vi "JitterVCOLO.vi"() -> ()   [LabVIEW 2009]
uses:
  <vilib>/Analysis/4window.llb/windowTd.ctl
  <vilib>/measure/maspectr.llb/FFT Spectrum (Mag-Phase) for 1 Chan.vi
  <vilib>/measure/maspectr.llb/FFT Power Spectrum for 1 Chan.vi
  <vilib>/measure/macond.llb/FIR Filter for 1 Chan.vi
  <vilib>/ptbypt/NI_PtbyPt.lvlib
  <vilib>/measure/NI_MAPro.lvlib
  <vilib>/Analysis/NI_AALPro.lvlib
  <vilib>/measure/NI_MABase.lvlib
panel:
  in  "FFT View":T1={"dB On (F)"=TRUE, "unwrap phase (F)"=FALSE, "convert to degree (F)"=FALSE}
  out "VCO Period":ext=1.25000000000000000005e-7 format="%#_6p"
  out "LO Period":ext=1.6666666666666666666e-7 format="%#_6p"
  out "Equivalent LO RMS time jitter":ext format="%#_6p"
  out "Equivalent VCO RMS time jitter":ext=1.9894367886486917747e-10 format="%#_6p"
  in  "Sampling rate and number of samples to generate":cluster{"Fs":dbl, "#s":dbl}={"Fs"=40000000.0, "#s"=400000.0} {"Fs" format="%.2p"}
  out "df (Hz)":dbl=100.0
  out "averages completed":dbl=1.0
  in  "averaging parameters":T2={"averaging mode"=enum."RMS averaging", "weighting mode"=enum."Exponential", "number of averages"=20} {"number of averages" min=1}
  in  "optional FIR filter specifications":T3={"PB Gain"=0.0, "SB Gain"=-300.0, "Scale"=TRUE, "Window"=enum."Flat Top"} {"SB Gain" format="%.2p"; "PB Gain" format="%.2p"}
  out "Computed Cycles":i32=400000
  in  "Low Side / High Side":bool
  out "Phase Noise":cluster{"f0":dbl, "df":dbl, "magnitude":dbl[]}(graph)={"f0"=0.0, "df"=100.0, "magnitude"=[]}
  out "RF input":cluster{"f0":dbl, "df":dbl, "magnitude":dbl[]}(graph)={"f0"=0.0, "df"=99.74415623924635, "magnitude"=[]}
  in  "VCO power (dBm)":dbl
  in  "LO power (dBm)":dbl
  in  "RMS Phase Jitter VCO (Radians)":ext=0.01
  in  "RMS Phase Jitter LO (Radians)":ext
  in  "VCO  Frequency":ext=8000000.0 format="%#.6p"
  in  "IF Frequency":ext=2000000.0 format="%#.6p"
  # "Phase noise power spectum (dBc), only good out to the lower PB of the FIR filter used after the\nI/Q downconversion from the intermediate frequency step"
  # "Nyquist demands that Fs > 2 * (2 * VCO - IF) for Low Side,\nand Fs > 2 * (2 * VCO + IF) for High Side"
  # "Enter the number of samples to generate here. This will affect your\nfrequency granularity. More samples, more granularity. df = Fs / (#s)"
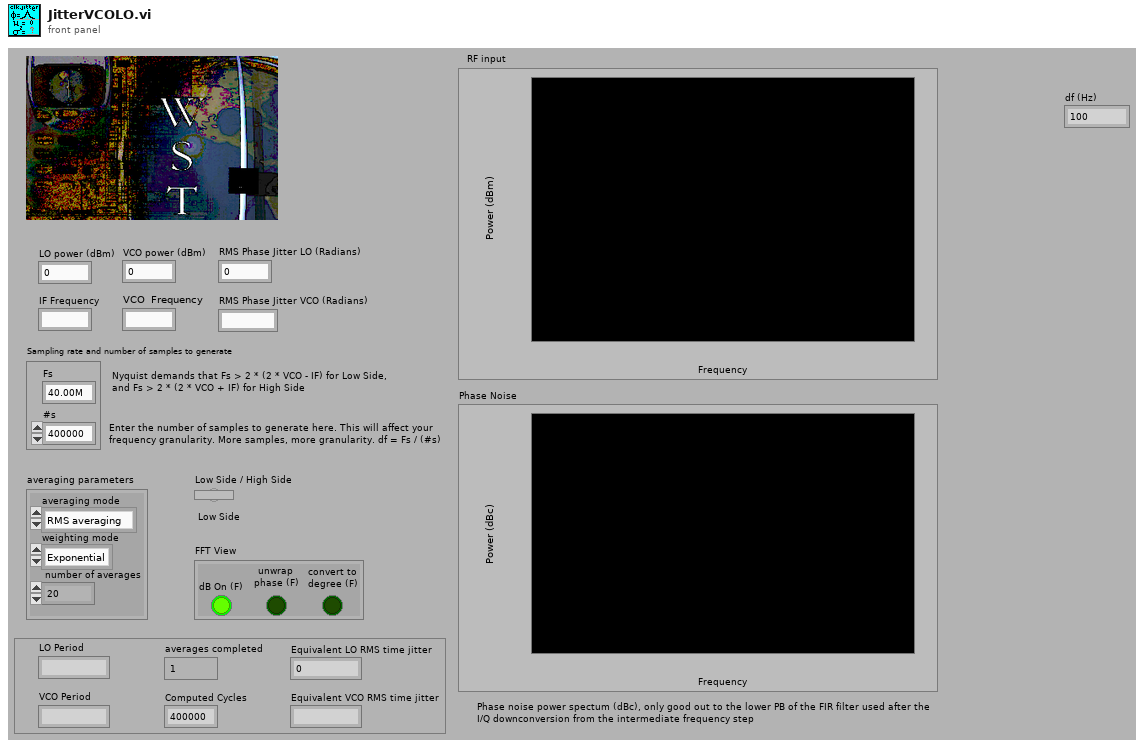
[diagram p1: front panel]
types:
  T1 = cluster{"dB On (F)":bool, "unwrap phase (F)":bool, "convert to degree (F)":bool}
  T2 = cluster{"averaging mode":enum16{"No averaging", "Vector averaging", "RMS averaging", "Peak hold"}, "weighting mode":enum16{"Linear", "Exponential"}, "number of averages":u32}
  T3 = cluster{"PB Gain":dbl, "SB Gain":dbl, "Scale":bool, "Window":enum16{"None", "Hanning", "Hamming", "Triangular", "Blackman", "Exact Blackman", "Blackman-Harris", "Kaiser-Bessel", "Flat Top"}}
  T4 = cluster{"Topology":enum16{"Off", "FIR by Specification", "Equi-ripple FIR", "Windowed FIR"}, "Type":enum16{"Lowpass", "Highpass", "Bandpass", "Bandstop"}, "#Taps":i32, "Lower PB":dbl, "Upper PB":dbl, "Lower SB":dbl, "Upper SB":dbl}
  T5 = enum16{"Off", "FIR by Specification", "Equi-ripple FIR", "Windowed FIR"}
  T6 = enum16{"Lowpass", "Highpass", "Bandpass", "Bandstop"}
  T7 = typedef "NI_AALPro.lvlib/windowTd.ctl" = u32
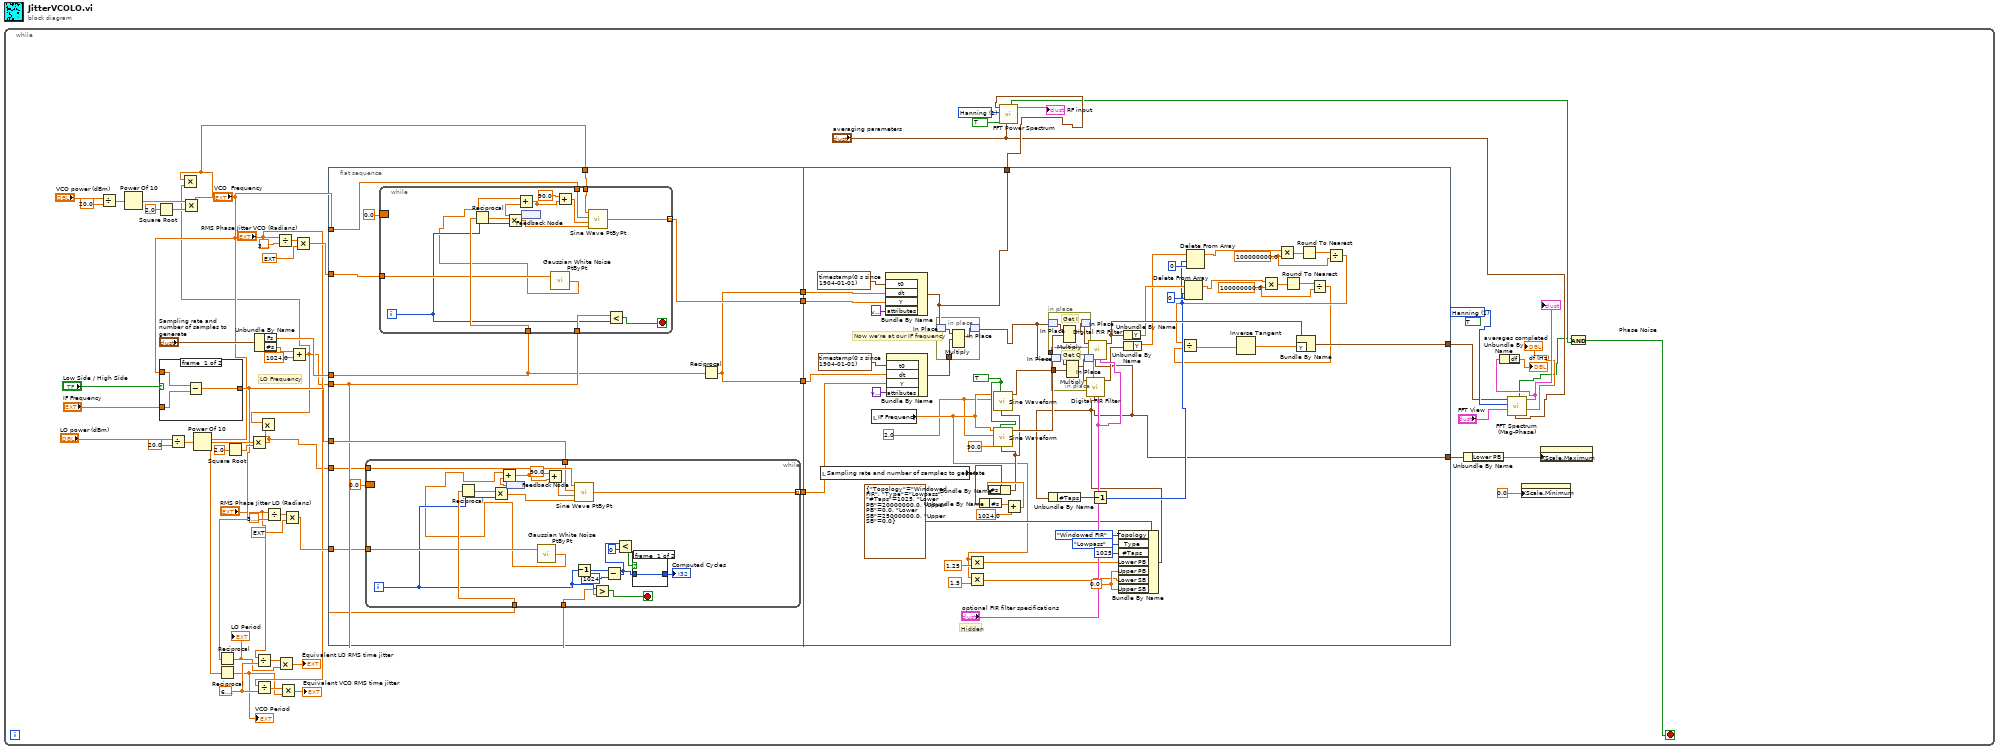
[diagram p0: block diagram]
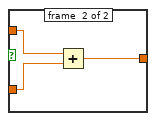
[diagram p2: hidden frame]
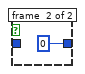
[diagram p3: hidden frame]
diagram:
  n1 = while {
    stop <- w31 stop-if-true
    w27 = 6.283185307179586
    w32 = T7 1 items=["Rectangle"=0, "Hanning"=1, "Hamming"=2, "Blackman-Harris"=3, "Exact Blackman"=4, "Blackman"=5, "Flat Top"=6, "4 Term B-Harris "=7, "7 Term B-Harris"=8, "Low Sidelobe"=9, "Blackman Nuttall"=11, "Triangle"=30, "Kaiser"=60, "Dolph-Chebyshev"=61, "Gaussian"=62] ("window")
    (unwired) TRUE ("dB On (F)")
    w9 = T7 1 items=["Rectangle"=0, "Hanning"=1, "Hamming"=2, "Blackman-Harris"=3, "Exact Blackman"=4, "Blackman"=5, "Flat Top"=6, "4 Term B-Harris "=7, "7 Term B-Harris"=8, "Low Sidelobe"=9, "Blackman Nuttall"=11, "Triangle"=30, "Kaiser"=60, "Dolph-Chebyshev"=61, "Gaussian"=62] ("window")
    # "LO Frequency"
    n2 = Divide(x="VCO power (dBm)", y=20.0) -> (x/y=w48:dbl)
    n3 = Power Of 10(x=w48) -> (10^x=w45:dbl)
    n4 = Square Root(x=2.0) -> (sqrt(x)=w46:dbl)
    n5 = case shown="False" "Low Side / High Side" {
      tunnel: "IF Frequency" -> [w63 w66]
      tunnel: "VCO  Frequency" -> [w64 w67]
      tunnel: [w62 w65] -> w26
      frame #0 {
        n6 = Subtract(x=w64, y=w63) -> (x-y=w62:ext)
      }
      frame #1 {
        n7 = Add(x=w67, y=w66) -> (x+y=w65:ext)
      }
    }
    n8 = Divide(x="LO power (dBm)", y=20.0) -> (x/y=w54:dbl)
    n9 = Multiply(x=w45, y=w46) -> (x*y=w13:dbl)
    n10 = Power Of 10(x=w54) -> (10^x=w51:dbl)
    n11 = Reciprocal(x=w26) -> (1/x=w18:ext)
    "LO Period" <- w18
    n12 = Reciprocal(x="VCO  Frequency") -> (1/x=w17:ext)
    "VCO Period" <- w17
    n13 = Square Root(x=2.0) -> (sqrt(x)=w52:dbl)
    n14 = Multiply(x=w51, y=w52) -> (x*y=w12:dbl)
    n15 = Unbundle By Name("Sampling rate and number of samples to generate") -> ("Fs"=w28:dbl, "#s"=w16:dbl)
    n16 = Divide(x="RMS Phase Jitter LO (Radians)", y=w27) -> (x/y=w23:ext)
    n17 = Divide(x="RMS Phase Jitter VCO (Radians)", y=w27) -> (x/y=w22:ext)
    n18 = Divide(x="RMS Phase Jitter LO (Radians)", y=3.141592653589793) -> (x/y=w38:ext)
    n19 = Divide(x="RMS Phase Jitter VCO (Radians)", y=3.141592653589793) -> (x/y=w41:ext)
    n20 = Multiply(x=w23, y=w18) -> (x*y=→"Equivalent LO RMS time jitter":ext)
    n21 = Multiply(x=w22, y=w17) -> (x*y=→"Equivalent VCO RMS time jitter":ext)
    n22 = Multiply(x=w38, y=ext 180.0) -> (x*y=w35:ext)
    n23 = Add(x=w16, y=1024.0) -> (x+y=w14:dbl)
    n24 = Multiply(x=w13, y=w14) -> ()  [unwired: 1 out]
    n25 = Multiply(x=w14, y=w12) -> ()  [unwired: 1 out]
    n26 = Multiply(x=w41, y=ext 180.0) -> (x*y=w39:ext)
    n27 = flat-sequence {
      tunnel: "VCO  Frequency" -> [w80]
      tunnel: w26 -> [w79]
      tunnel: w14 -> [w78]
      tunnel: w28 -> [w77]
      tunnel: [w75] -> w61
      tunnel: [w76] -> w60
      tunnel: [w75] -> w59
      tunnel: [w74] -> w58
      tunnel: w35 -> [w73]
      tunnel: w39 -> [w72]
      tunnel: w12 -> [w71]
      tunnel: w13 -> [w70]
      tunnel: w61 -> [w173]
      tunnel: w60 -> [w172]
      tunnel: w59 -> [w170]
      tunnel: w58 -> [w169]
      tunnel: [w142] -> w7
      tunnel: [w141] -> w11
      tunnel: [w133] -> w30
      frame #0 {
        n28 = while {
          tunnel: w77 -> [w101]
          tunnel: [w99] -> w74 mode=indexing
          tunnel: w78 -> [w92]
          tunnel: w79 -> [w94]
          tunnel: w73 -> [w97]
          tunnel: w71 -> [w96]
          border: 0.0 -> [_]
          i -> [w91]
          stop <- w98 stop-if-true
          n29 = Reciprocal(x=w101) -> (1/x=w95:dbl)
          n30 = Multiply(x=w95, y=w91) -> (x*y=w100:dbl)
          n31 = feedback #1() -> (w88:dbl)
          n32 = call <vilib>:"Gaussian White Noise PtByPt.vi"("standard deviation"=w97) -> ("Gaussian white noise"=w90:dbl)  [unwired: 2 in]
          n33 = Add(x=w90, y=w88) -> (x+y=w87:dbl)
          n34 = Add(x=90.0, y=w87) -> (x+y=w89:dbl)
          n35 = call <vilib>:"Sine Wave PtByPt.vi"("time"=w100, "phase"=w89, "frequency"=w94, "amplitude"=w96) -> ("sine wave"=w99:dbl)
          n36 = Decrement(x=w91) -> (x-1=w86:i32)
          n37 = Greater?(x=w91, y=w92) -> (0:w98:bool)
          n38 = Subtract(x=w86, y=1024) -> (x-y=w81:i32)
          n39 = Less?(x=w81, y=0) -> (x < y?=w83:bool)
          n40 = case shown="False" w83 {
            tunnel: [w102 0] -> w82
            tunnel: w81 -> [w102 _]
            frame #0 {
            }
            frame #1 {
            }
          }
          "Computed Cycles" <- w82
        }
        n41 = while {
          tunnel: w77 -> [w118]
          tunnel: [w116] -> w76 mode=indexing
          tunnel: w78 -> [w109]
          tunnel: w80 -> [w111]
          tunnel: w72 -> [w114]
          tunnel: w70 -> [w113]
          border: 0.0 -> [_]
          i -> [w108]
          stop <- w115 stop-if-true
          n42 = Reciprocal(x=w118) -> (1/x=w117:dbl)
          n43 = Multiply(x=w117, y=w108) -> (x*y=w112:dbl)
          n44 = feedback #2() -> (w105:dbl)
          n45 = call <vilib>:"Gaussian White Noise PtByPt.vi"("standard deviation"=w114) -> ("Gaussian white noise"=w107:dbl)  [unwired: 2 in]
          n46 = Add(x=w107, y=w105) -> (x+y=w104:dbl)
          n47 = Add(x=90.0, y=w104) -> (x+y=w106:dbl)
          n48 = call <vilib>:"Sine Wave PtByPt.vi"("time"=w112, "phase"=w106, "frequency"=w111, "amplitude"=w113) -> ("sine wave"=w116:dbl)
          n49 = Less?(x=w109, y=w108) -> (x < y?=w115:bool)
        }
        n50 = Reciprocal(x=w77) -> (1/x=w75:dbl)
      }
      frame #1 {
        w139 = 0.0 ("Lower SB")
        w140 = TRUE ("reset signal")
        w145 = 100000000.0 ("y")
        w147 = 100000000.0 ("y")
        w119 = 2.0 ("amplitude")
        # "Hidden"
        # "Get Q"
        # "Get I"
        # "Now we're at our IF frequency"
        n51 = local read "Sampling rate and number of samples to generate"() -> (w129:cluster{"Fs":dbl, "#s":dbl})
        n52 = local read "IF Frequency"() -> (w124:ext)
        n53 = Bundle By Name("t0"=timestamp(0 s since 1904-01-01), "dt"=w173, "Y"=w172, "attributes"=variant) -> (w141:waveform(dbl))  [unwired: 1 in]
        n54 = Bundle By Name("t0"=timestamp(0 s since 1904-01-01), "dt"=w170, "Y"=w169, "attributes"=variant) -> (w166:waveform(dbl))  [unwired: 1 in]
        n55 = in-place {
          in-place-border: w166 -> [w177]
          n56 = in-place-match #3(w141) -> (w175:waveform(dbl))
          n57 = Multiply(1:w177, 2:w175) -> (0:w176:waveform(dbl))  [unwired: 1 in, 1 out]
          n58 = in-place-match #3(w176) -> (w161:waveform(dbl))
        }
        n59 = Multiply(x=w124, y=1.25) -> (x*y=w126:ext)
        n60 = Multiply(x=w124, y=1.5) -> (x*y=w125:ext)
        n61 = Unbundle By Name(w129) -> ("#s"=w132:dbl)
        n62 = Add(x=w132, y=1024.0) -> (x+y=w130:dbl)
        n63 = Bundle By Name(cluster=w129, "#s"=w130) -> (w128:cluster{"Fs":dbl, "#s":dbl})
        n64 = call <vilib>:"Sine Waveform.vi"("sampling info"=w128, "reset signal"=w140, "amplitude"=w119, "frequency"=w124) -> ("signal out"=w165:waveform(dbl))  [unwired: 6 in, 1 out]
        n65 = call <vilib>:"Sine Waveform.vi"("sampling info"=w128, "reset signal"=w140, "phase"=90.0, "amplitude"=w119, "frequency"=w124) -> ("signal out"=w164:waveform(dbl))  [unwired: 5 in, 1 out]
        n66 = in-place {
          in-place-border: w164 -> [w180]
          n67 = in-place-match #4(w161) -> (w179:waveform(dbl))
          n68 = Multiply(1:w180, 2:w179) -> (0:w178:waveform(dbl))  [unwired: 1 in, 1 out]
          n69 = in-place-match #4(w178) -> (w160:waveform(dbl))
        }
        n70 = in-place {
          in-place-border: w165 -> [w183]
          n71 = in-place-match #5(w161) -> (w182:waveform(dbl))
          n72 = Multiply(1:w183, 2:w182) -> (0:w181:waveform(dbl))  [unwired: 1 in, 1 out]
          n73 = in-place-match #5(w181) -> (w159:waveform(dbl))
        }
        n74 = Bundle By Name(cluster=T4 {"Topology"=enum."Windowed FIR", "Type"=enum."Lowpass", "#Taps"=1025, "Lower PB"=20000000.0, "Upper PB"=0.0, "Lower SB"=25000000.0, "Upper SB"=0.0} ("FIR filter specifications"), "Topology"=T5."Windowed FIR", "Type"=T6."Lowpass", "#Taps"=1025, "Lower PB"=w126, "Upper PB"=w139, "Lower SB"=w125, "Upper SB"=w139) -> (w133:T4)
        n75 = Unbundle By Name(w133) -> ("#Taps"=w155:i32)
        n76 = call-poly <vilib>:"Digital FIR Filter.vi"("optional FIR filter specifications"="optional FIR filter specifications", "FIR filter specifications"=w133, "signal in"=w159) -> ("signal out"=w157:waveform(dbl))  [unwired: 6 in, 2 out]
        n77 = call-poly <vilib>:"Digital FIR Filter.vi"("optional FIR filter specifications"="optional FIR filter specifications", "FIR filter specifications"=w133, "signal in"=w160) -> ("signal out"=w158:waveform(dbl))  [unwired: 6 in, 2 out]
        n78 = Decrement(x=w155) -> (x-1=w151:i32)
        n79 = Unbundle By Name(w158) -> ("Y"=w156:dbl[])
        n80 = Unbundle By Name(w157) -> ("Y"=w152:dbl[])
        n81 = Delete From Array(array=w156, length=w151, index=0) -> (array with subset deleted=w143:dbl[])  [unwired: 1 out]
        n82 = Delete From Array(array=w152, length=w151, index=0) -> (array with subset deleted=w150:dbl[])  [unwired: 1 out]
        n83 = Multiply(x=w143, y=w145) -> (x*y=w144:dbl[])
        n84 = Multiply(x=w150, y=w147) -> (x*y=w149:dbl[])
        n85 = Round To Nearest(number=w144) -> (nearest integer value=w146:dbl[])
        n86 = Round To Nearest(number=w149) -> (nearest integer value=w148:dbl[])
        n87 = Divide(x=w146, y=w145) -> (x/y=w121:dbl[])
        n88 = Divide(x=w148, y=w147) -> (x/y=w122:dbl[])
        n89 = Divide(x=w122, y=w121) -> (x/y=w120:dbl[])
        n90 = Inverse Tangent(1:w120) -> (0:w123:dbl[])
        n91 = Bundle By Name(cluster=w158, "Y"=w123) -> (w142:waveform(dbl))
      }
    }
    n92 = call-poly <vilib>:"FFT Power Spectrum.vi"("averaging parameters"="averaging parameters", "dB On (F)"=TRUE, "window"=w32, "time signal"=w11) -> ("power spectrum"=→"RF input":cluster{"f0":dbl, "df":dbl, "magnitude":dbl[]}, "averaging done"=w2:bool)  [unwired: 4 in, 2 out]
    n93 = Unbundle By Name(w30) -> ("Lower PB"=w10:dbl)
    n94 = call-poly <vilib>:"FFT Spectrum (Mag-Phase).vi"("averaging parameters"="averaging parameters", "view"="FFT View", "window"=w9, "time signal"=w7) -> ("averages completed"=→"averages completed":dbl, "magnitude"=w5:cluster{"f0":dbl, "df":dbl, "magnitude":dbl[]}, "averaging done"=w1:bool)  [unwired: 3 in, 2 out]
    "Phase Noise" <- w5
    n95 = Unbundle By Name(w5) -> ("df"=→"df (Hz)":dbl)
    n96 = property on="Phase Noise" class="WFGraph (strict)"("XScale.Minimum"=0.0 ("X Scale.Range:Minimum")) -> ()  [unwired: 2 in, 2 out]
    n97 = property on="Phase Noise" class="WFGraph (strict)"("XScale.Maximum"=w10) -> ()  [unwired: 2 in, 2 out]
    n98 = And(x=w1, y=w2) -> (x .and. y?=w31:bool)
  }
